vi "LEBITplc.CreateMinAndMaxSetValues.vi"(1 "Info Array from DB":string[][](array[string])) -> (0 "Min & Max Array":string[][](array[string]))   [LabVIEW 2014, in "LEBITplc.lvlib"]
uses:
  LEBITplc.lvlib
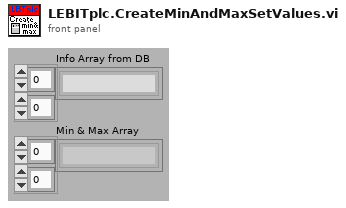
[diagram p1: front panel]
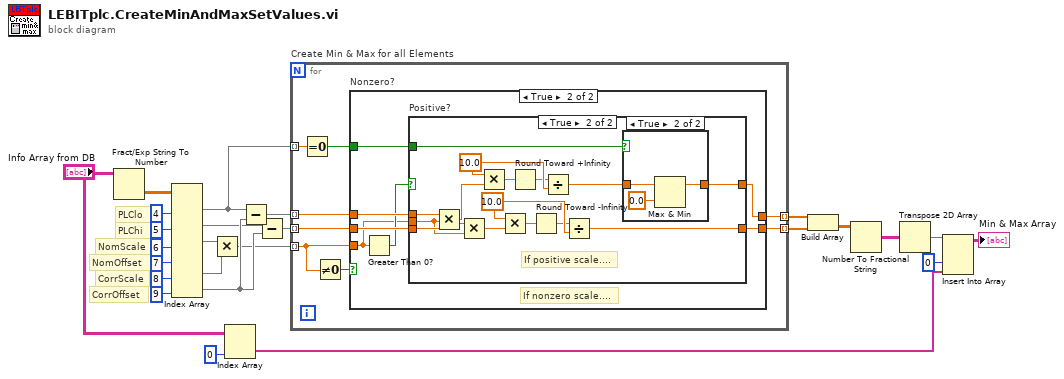
[diagram p0: block diagram]
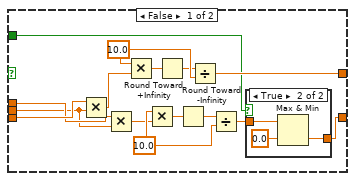
[diagram p3: hidden frame]
diagram:
  # "CorrOffset"
  # "CorrScale"
  # "NomOffset"
  # "NomScale"
  # "PLChi"
  # "PLClo"
  n1 = Fract/Exp String To Number(string="Info Array from DB") -> (number=w25:dbl[][])  [unwired: 3 in, 1 out]
  n2 = Index Array(array=w25, index (col) #1=4 ("disabled index (col)"), index (col) #2=5 ("index (col)"), index (col) #3=6 ("index (col)"), index (col) #4=7 ("index (col)"), index (col) #5=8 ("index (col)"), index (col) #6=9 ("index (col)")) -> (element #1=w7:dbl[], element #2=w8:dbl[], element #3=w18:dbl[], element #5=w17:dbl[], element #6=w14:dbl[])  [unwired: 6 in, 1 out]
  n3 = Multiply(x=w18, y=w17) -> (x*y=w11:dbl[])
  n4 = Index Array(array="Info Array from DB", index (col)=0 ("disabled index (col)")) -> (element=w1:string[])  [unwired: 1 in]
  n5 = Subtract(x=w7, y=w14) -> (x-y=w16:dbl[])
  n6 = Subtract(x=w8, y=w14) -> (x-y=w15:dbl[])
  n7 = for "Create Min & Max for all Elements" {
    tunnel: w16 -> [w33] mode=indexing
    tunnel: w15 -> [w32] mode=indexing
    tunnel: [w31] -> w13 mode=indexing
    tunnel: [w30] -> w12 mode=indexing
    tunnel: w11 -> [w28] mode=indexing
    tunnel: w7 -> [w27] mode=indexing
    n8 = Equal To 0?(x=w27) -> (x = 0?=w26:bool)
    n9 = Not Equal To 0?(x=w28) -> (x != 0?=w29:bool)
    n10 = case "Nonzero?" shown="True" w29 {
      tunnel: w33 -> [w35 w42]
      tunnel: w32 -> [w34 w41]
      tunnel: [w35 w40] -> w31
      tunnel: [w34 w39] -> w30
      tunnel: w28 -> [_ w37]
      tunnel: w26 -> [_ w36]
      frame False {
      }
      frame True {
        # "If nonzero scale...."
        n11 = Greater Than 0?(x=w37) -> (x > 0?=w38:bool)
        n12 = case "Positive?" shown="True" w38 {
          tunnel: w42 -> [w48 w76]
          tunnel: w41 -> [w49 w75]
          tunnel: [w47 w63] -> w40
          tunnel: [w44 w62] -> w39
          tunnel: w37 -> [w46 w66]
          tunnel: w36 -> [w43 w65]
          frame False {
            w53 = 10.0
            w57 = 10.0
            n13 = Multiply(x=w49, y=w46) -> (x*y=w54:dbl)
            n14 = Multiply(x=w48, y=w46) -> (x*y=w50:dbl)
            n15 = Multiply(x=w57, y=w54) -> (x*y=w56:dbl)
            n16 = Multiply(x=w53, y=w50) -> (x*y=w52:dbl)
            n17 = Round Toward +Infinity(x=w56) -> (ceil(x): smallest int >= x=w55:dbl)
            n18 = Round Toward -Infinity(1:w52) -> (0:w51:dbl)
            n19 = Divide(x=w55, y=w57) -> (x/y=w47:dbl)
            n20 = Divide(x=w51, y=w53) -> (x/y=w45:dbl)
            n21 = case shown="True" w43 {
              tunnel: w45 -> [w58 w61]
              tunnel: [w58 w59] -> w44
              frame False {
              }
              frame True {
                n22 = Max & Min(x=w61, y=0.0) -> (min(x,y)=w59:dbl)  [unwired: 1 out]
              }
            }
          }
          frame True {
            w70 = 10.0
            w74 = 10.0
            # "If positive scale...."
            n23 = Multiply(x=w76, y=w66) -> (x*y=w71:dbl)
            n24 = Multiply(x=w75, y=w66) -> (x*y=w67:dbl)
            n25 = Multiply(x=w74, y=w71) -> (x*y=w73:dbl)
            n26 = Multiply(x=w70, y=w67) -> (x*y=w69:dbl)
            n27 = Round Toward +Infinity(x=w73) -> (ceil(x): smallest int >= x=w72:dbl)
            n28 = Round Toward -Infinity(1:w69) -> (0:w68:dbl)
            n29 = Divide(x=w72, y=w74) -> (x/y=w64:dbl)
            n30 = Divide(x=w68, y=w70) -> (x/y=w62:dbl)
            n31 = case shown="True" w65 {
              tunnel: w64 -> [w77 w80]
              tunnel: [w77 w78] -> w63
              frame False {
              }
              frame True {
                n32 = Max & Min(x=w80, y=0.0) -> (max(x,y)=w78:dbl)  [unwired: 1 out]
              }
            }
          }
        }
      }
    }
  }
  n33 = Build Array(w13, w12) -> (w10:dbl[][])
  n34 = Number To Fractional String(number=w10) -> (F-format string=w9:string[][])  [unwired: 3 in]
  n35 = Transpose 2D Array(2D array=w9) -> (transposed array=w3:string[][])
  n36 = Insert Into Array(array=w3, index (col)=0 ("disabled index (col)"), new element=w1) -> (→"Min & Max Array":string[][])  [unwired: 1 in]
